vi "Distribute - Horizontal Compress.vi"(6 "Variant in":variant, 7 "Shift Pressed?":bool, 8 "error in (no error)":errorcluster, 10 "QD Combo Box Ref":refnum<vi>, 11 "QD Launch VI Ref":refnum<vi>) -> (0 "error out":errorcluster, 4 "Variant out":variant)   [LabVIEW 2017, in "Align and Distribute.lvlib"]
doc: "Compresses the selected front panel objects horizontally by removing the gaps between them."
uses:
  Align and Distribute.lvlib
panel:
  # "Do not change the connector pane of this VI."
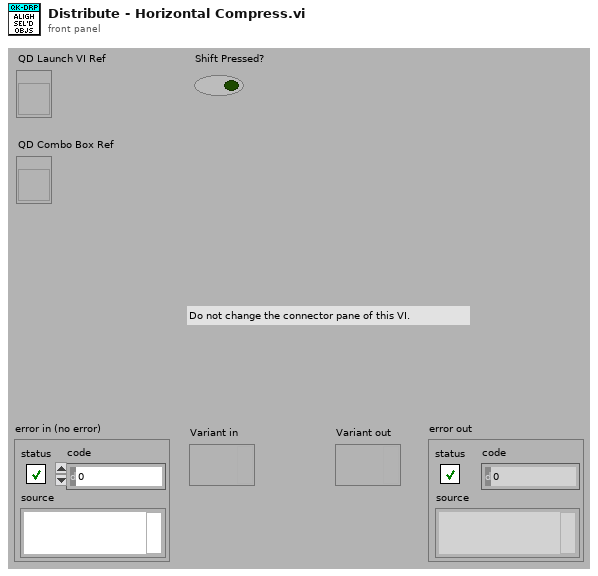
[diagram p1: front panel]
types:
  T1 = enum32{"Top Edges", "Vertical Centers", "Bottom Edges", "Vertical Gap", "Vertical Compress", "Left Edges", "Horizontal Centers", "Right Edges", "Horizontal Gap", "Horizontal Compress"}
  T2 = enum32{"Top Edges", "Vertical Centers", "Bottom Edges", "Left Edges", "Horizontal Centers", "Right Edges"}
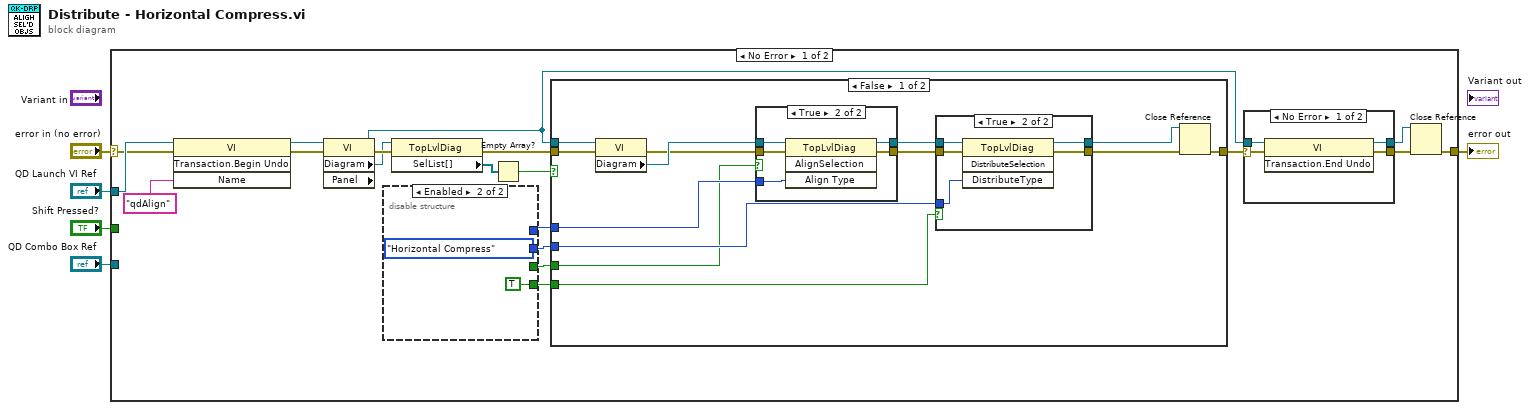
[diagram p0: block diagram]
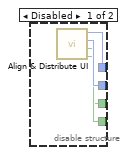
[diagram p2: hidden frame]
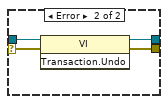
[diagram p3: hidden frame]
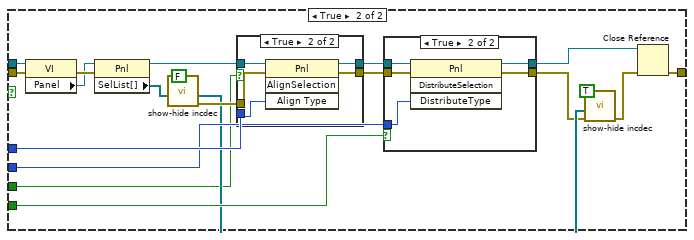
[diagram p6: hidden frame]
diagram:
  n1 = case shown="No Error" "error in (no error)" {
    selector: "error in (no error)" -> [w17 w100]
    tunnel: [w20 w100] -> w4
    tunnel: "QD Launch VI Ref" -> [w19 _]
    tunnel: "Shift Pressed?" -> [_ _]
    tunnel: "QD Combo Box Ref" -> [_ _]
    frame No Error {
      n2 = invoke class="VI" method="Transaction.Begin Undo"(reference=w19, error in=w17, "Name"="qdAlign") -> (reference out=w18:refnum<vi>, error out=w16:errorcluster)  [unwired: 1 in, 2 out]
      n3 = property class="VI" props=["Diagram", "Panel"](reference=w18, error in=w16) -> (reference out=w13:refnum<vi>, error out=w24:errorcluster, "Diagram"=w23:refnum<vi>)  [unwired: 1 out]
      n4 = disable-structure shown="Enabled" {
        disable-tunnel: [w28 _] -> w11
        disable-tunnel: [w27 T1."Horizontal Compress" ("Distribute Type")] -> w10
        disable-tunnel: [w26 TRUE ("Distribute Type valid?")] -> w7
        disable-tunnel: [w25 _] -> w6
        frame Disabled {
          n5 = call "Align & Distribute UI.vi"() -> ("Distribute Type valid?"=w26:bool, "Align Type valid?"=w25:bool, "Distribute Type"=w27:T1, "Align Type"=w28:T2)  [unwired: 8 in]
        }
        frame Enabled {
        }
      }
      n6 = property class="TopLvlDiag"(reference=w23, error in=w24) -> (error out=w21:errorcluster, "SelList[]"=w8:refnum<vi>[])  [unwired: 1 out]
      n7 = Empty Array?(array=w8) -> (empty?=w22:bool)
      n8 = case shown="False" w22 {
        tunnel: w21 -> [w50 w85]
        tunnel: w13 -> [w49 w84]
        tunnel: [w51 w83] -> w9
        tunnel: w11 -> [w46 w82]
        tunnel: w7 -> [w41 w78]
        tunnel: w10 -> [w40 w77]
        tunnel: w6 -> [w39 w66]
        frame False {
          n9 = property class="VI"(reference=w49, error in=w50) -> (error out=w47:errorcluster, "Diagram"=w48:refnum<vi>)  [unwired: 1 out]
          n10 = case shown="True" w39 {
            tunnel: w48 -> [w53 w58]
            tunnel: w47 -> [w52 w57]
            tunnel: w46 -> [_ w56]
            tunnel: [w52 w55] -> w45
            tunnel: [w53 w54] -> w44
            frame False {
            }
            frame True {
              n11 = invoke class="TopLvlDiag" method="AlignSelection"(reference=w58, error in=w57, "Align Type"=w56) -> (reference out=w54:refnum<vi>, error out=w55:errorcluster)  [unwired: 1 in, 2 out]
            }
          }
          n12 = case shown="True" w41 {
            tunnel: w45 -> [w60 w65]
            tunnel: w44 -> [w59 w64]
            tunnel: [w59 w63] -> w43
            tunnel: [w60 w62] -> w42
            tunnel: w40 -> [_ w61]
            frame False {
            }
            frame True {
              n13 = invoke class="TopLvlDiag" method="DistributeSelection"(reference=w64, error in=w65, "DistributeType"=w61) -> (reference out=w63:refnum<vi>, error out=w62:errorcluster)  [unwired: 1 in, 2 out]
            }
          }
          n14 = Close Reference(reference=w43, error in (no error)=w42) -> (error out=w51:errorcluster)
        }
        frame True {
          n15 = property class="VI"(reference=w84, error in=w85) -> (error out=w74:errorcluster, "Panel"=w73:refnum<vi>)  [unwired: 1 out]
          n16 = property class="Pnl"(reference=w73, error in=w74) -> (reference out=w72:refnum<vi>, "SelList[]"=w75:refnum<vi>[])  [unwired: 1 out]
          n17 = call "show-hide incdec.vi"("Show?"=FALSE, "SelList[]"=w75) -> ("error out"=w71:errorcluster, "SelList[] out"=w69:refnum<vi>[])  [unwired: 8 in]
          n18 = case shown="True" w66 {
            tunnel: w82 -> [_ w92]
            tunnel: [w86 w91] -> w81
            tunnel: [w87 w90] -> w80
            tunnel: w72 -> [w87 w89]
            tunnel: w71 -> [w86 w88]
            frame False {
            }
            frame True {
              n19 = invoke class="Pnl" method="AlignSelection"(reference=w89, error in=w88, "Align Type"=w92) -> (reference out=w90:refnum<vi>, error out=w91:errorcluster)  [unwired: 1 in, 2 out]
            }
          }
          n20 = case shown="True" w78 {
            tunnel: w81 -> [w94 w99]
            tunnel: w80 -> [w93 w98]
            tunnel: [w93 w97] -> w79
            tunnel: [w94 w96] -> w68
            tunnel: w77 -> [_ w95]
            frame False {
            }
            frame True {
              n21 = invoke class="Pnl" method="DistributeSelection"(reference=w98, error in=w99, "DistributeType"=w95) -> (reference out=w97:refnum<vi>, error out=w96:errorcluster)  [unwired: 1 in, 2 out]
            }
          }
          n22 = call "show-hide incdec.vi"("Show?"=TRUE, "error in"=w68, "SelList[]"=w69) -> ("error out"=w67:errorcluster)  [unwired: 7 in, 1 out]
          n23 = Close Reference(reference=w79, error in (no error)=w67) -> (error out=w83:errorcluster)
        }
      }
      n24 = case shown="No Error" w9 {
        selector: w9 -> [w31 w38]
        tunnel: [w34 w37] -> w14
        tunnel: w13 -> [w33 w36]
        tunnel: [w32 w35] -> w12
        frame No Error {
          n25 = invoke class="VI" method="Transaction.End Undo"(reference=w33, error in=w31) -> (reference out=w32:refnum<vi>, error out=w34:errorcluster)  [unwired: 1 in, 1 out]
        }
        frame Error {
          n26 = invoke class="VI" method="Transaction.Undo"(reference=w36, error in=w38) -> (reference out=w35:refnum<vi>, error out=w37:errorcluster)  [unwired: 1 in, 1 out]
        }
      }
      n27 = Close Reference(reference=w12, error in (no error)=w14) -> (error out=w20:errorcluster)
    }
    frame Error {
    }
  }
  "error out" <- w4
